vi "Manually Configure Acceleration Offset.vi"(0 "VISA resource name":refnum<visa-resource-name>, 5 "X Axis Accelerometer Offset (0 m/s^2)":sgl, 7 "Y Axis Accelerometer Offset  (0 m/s^2)":sgl, 9 "Z Axis Accelerometer Offset  (0 m/s^2)":sgl, 11 "error in (no error)":errorcluster) -> (4 "VISA resource name out":refnum<visa-resource-name>, 15 "error out":errorcluster)   [LabVIEW 2012, in "MicroStrain 3DM-GXx.lvlib"]
doc: "The specified values of AccelOffsetX, AccelOffsetY, and AccelOffsetZ (m/s^2) will be subtracted from all subsequent measurements of acceleration.\n\nThe above values will be stored in RAM. To save the values in non-volatile memory use the 'Transfer Calibration To EEPROM' VI after this VI."
uses:
  <instrlib>/MicroStrain 3DM-GXx/MicroStrain 3DM-GXx.lvlib
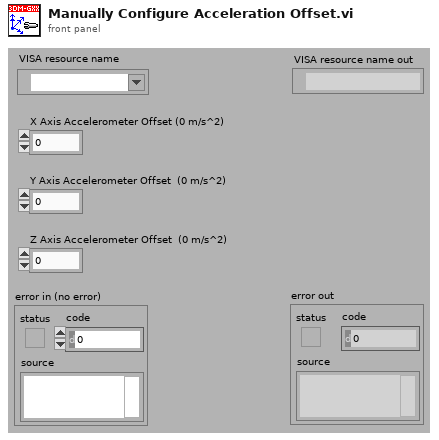
[diagram p1: front panel]
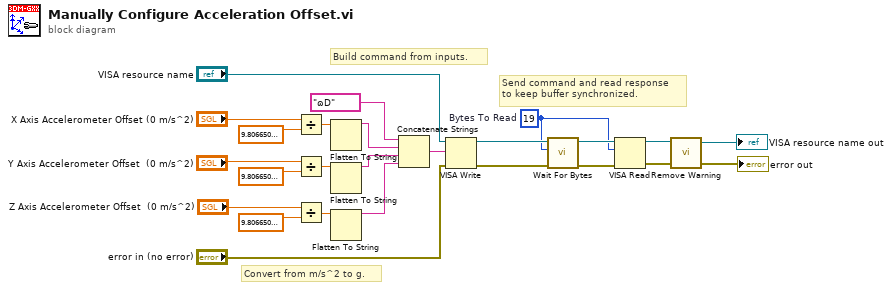
[diagram p0: block diagram]
diagram:
  w14 = u32 19  # Bytes To Read
  # "Convert from m/s^2 to g."
  # "Send command and read response\nto keep buffer synchronized."
  # "Build command from inputs."
  n1 = Divide(x="X Axis Accelerometer Offset (0 m/s^2)", y=sgl 9.80665) -> (x/y=w7:sgl)
  n2 = Divide(x="Y Axis Accelerometer Offset  (0 m/s^2)", y=sgl 9.80665) -> (x/y=w6:sgl)
  n3 = Divide(x="Z Axis Accelerometer Offset  (0 m/s^2)", y=sgl 9.80665) -> (x/y=w5:sgl)
  n4 = Flatten To String(anything=w7) -> (data string=w24:string)  [unwired: 3 in, 2 out]
  n5 = Flatten To String(anything=w6) -> (data string=w23:string)  [unwired: 3 in, 2 out]
  n6 = Flatten To String(anything=w5) -> (data string=w22:string)  [unwired: 3 in, 2 out]
  n7 = Concatenate Strings("ɷD", w24, w23, w22) -> (w21:string)
  n8 = VISA Write(VISA resource name="VISA resource name", write buffer=w21, error in (no error)="error in (no error)") -> (VISA resource name out=w18:refnum<visa-resource-name>, error out=w17:errorcluster)  [unwired: 1 out]
  n9 = call <instrlib>:"Wait For Bytes.vi"("error in (no error)"=w17, "Bytes To Read (0)"=w14, "VISA resource name"=w18) -> ("error out"=w15:errorcluster, "VISA resource name out"=w16:refnum<visa-resource-name>)  [unwired: 7 in]
  n10 = VISA Read(VISA resource name=w16, byte count=w14, error in (no error)=w15) -> (VISA resource name out=w4:refnum<visa-resource-name>, error out=w3:errorcluster)  [unwired: 2 out]
  n11 = call <instrlib>:"Remove Warning.vi"("error in (no error)"=w3, "VISA resource name"=w4) -> ("error out"=→"error out":errorcluster, "VISA resource name out"=→"VISA resource name out":refnum<visa-resource-name>)  [unwired: 2 in]
